vi "setpiece.vi"(1 "group":i32, 2 "piece":i32) -> (0 "Ring":u16(ring))   [LabVIEW 2024]
panel:
  out "all piece":u16(ring)
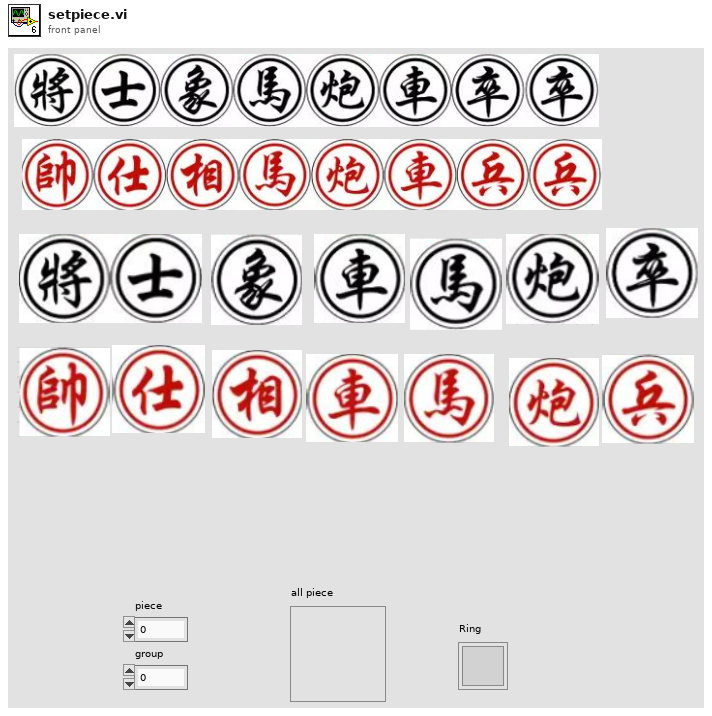
[diagram p1: front panel]
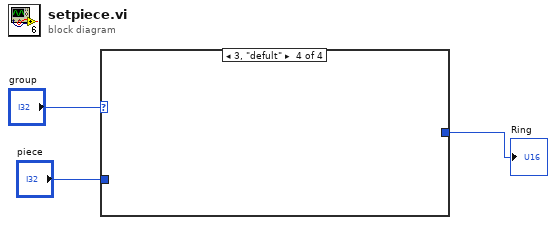
[diagram p0: block diagram]
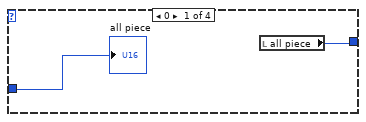
[diagram p2: hidden frame]
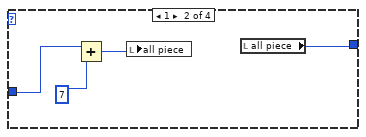
[diagram p3: hidden frame]
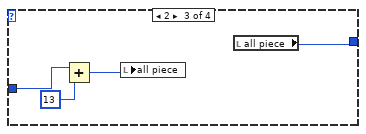
[diagram p4: hidden frame]
diagram:
  n1 = case shown="3, \"defult\"" "group" {
    tunnel: "piece" -> [w5 w9 w13 _]
    tunnel: [w4 w6 w10 _] -> w2
    frame 0 {
      n2 = local read "all piece"() -> (w4:u16)
      "all piece" <- w5
    }
    frame 1 {
      n3 = Add(x=w9, y=7) -> (x+y=w7:i32)
      n4 = local write "all piece"(w7) -> ()
      n5 = local read "all piece"() -> (w6:u16)
    }
    frame 2 {
      n6 = Add(x=w13, y=13) -> (x+y=w11:i32)
      n7 = local write "all piece"(w11) -> ()
      n8 = local read "all piece"() -> (w10:u16)
    }
    frame 3, 0 {
    }
  }
  "Ring" <- w2
